vi "GET HARDWARE REFS CLUSTER.vi"(11 "HARDWARE cluster":T22 {"MOTORS"."Motor Controller" items=["SPARK", "Existing", "SD540", "TALON SRX", "VICTOR SP", "TALON SR", "JAGUAR", "VICTOR"]; "AIR"."PRESSURE"."warning HIGH" format="%.2f"; "AIR"."PRESSURE"."warning LOW" format="%.2f"; "AIR"."PRESSURE"."nominal value" format="%.2f"; "DRIVE MOTORS"."Motor Controller" items=["SPARK", "Existing", "SD540", "TALON SRX", "VICTOR SP", "TALON SR", "JAGUAR", "VICTOR"]}) -> (1 "REF OUTPUT":cluster{T12[], T16[], T17[]}, 2 "REF INPUT":cluster{T1[], T3[], T7[], T9[], T10[]}, 3 "REF DRIVE JOYSTICK":T21)   [LabVIEW 2017]
uses:
  Controls/def HARDWARE CTRL info.ctl
  Controls/def MOTOR info.ctl
  Controls/ctrl MOTOR CTRLR SELECT.ctl
  <vilib>/Rock Robotics/SystemInterfaces/DIO/FPGA_DIOPWMChannel.ctl
  Controls/def USER CONTROL info.ctl
  <vilib>/Rock Robotics/WPI/Joystick/WPI_JoystickDeviceEnum.ctl
  Controls/def ENCODER info.ctl
  <vilib>/Rock Robotics/SystemInterfaces/DIO/FPGA_DIOChannel.ctl
  <vilib>/Rock Robotics/WPI/Encoder/WPI_EncoderType.ctl
  Controls/def GYRO info.ctl
  <vilib>/Rock Robotics/SystemInterfaces/spilib/spi_bus.ctl
  Controls/ctrl ANALOG CHANNEL SELECT.ctl
  Controls/def AIR PRESSURE info.ctl
  <vilib>/Rock Robotics/SystemInterfaces/AI/FPGA_AIChannel.ctl
  Controls/def COMPRESSOR info.ctl
  Controls/def SOLENOID info.ctl
  <vilib>/Rock Robotics/WPI/Solenoid/WPI_SolenoidChannel.ctl
  <vilib>/Rock Robotics/WPI/Solenoid/WPI_SolenoidValue.ctl
  Controls/def SERVO info.ctl
  Controls/def SONAR info.ctl
  Controls/ctrl SONAR DEVICE SELECT.ctl
  <vilib>/Rock Robotics/WPI/Ultrasonic/WPI_UltrasonicRangeUnits.ctl
  Controls/def RELAY info.ctl
  <vilib>/Rock Robotics/SystemInterfaces/DIO/FPGA_DIORelayChannel.ctl
  <vilib>/Rock Robotics/WPI/Relay/WPI_RelayDirection.ctl
  <vilib>/Rock Robotics/WPI/Relay/WPI_RelayValue.ctl
  Controls/def LIMIT SWITCH info.ctl
  <vilib>/Rock Robotics/WPI/Joystick/WPI_JoystickDevRef.ctl
  <vilib>/Rock Robotics/WPI/RobotDrive/WPI_RobotDriveDevRef.ctl
  <vilib>/Rock Robotics/WPI/MotorControl/WPI_MotorControlDeviceRef.ctl
  <vilib>/Rock Robotics/WPI/MotorControl/WPI_MotorControlType.ctl
  <vilib>/Rock Robotics/WPI/PWM/WPI_PWMDeadband.ctl
  <vilib>/Rock Robotics/WPI/PWM/Servo/WPI_ServoDeviceRef.ctl
  <vilib>/Rock Robotics/WPI/Relay/WPI_RelayDevRef.ctl
  <vilib>/Rock Robotics/WPI/Encoder/WPI_EncoderDevRef.ctl
  <vilib>/Rock Robotics/SystemInterfaces/Encoder/FPGA_EncoderIdx.ctl
  <vilib>/Rock Robotics/SystemInterfaces/Counter/FPGA_CounterCtrSystemIndex.ctl
  <vilib>/Rock Robotics/WPI/Ultrasonic/WPI_UltrasonicDeviceRef.ctl
  <vilib>/Rock Robotics/WPI/Switch/WPI_SwitchDevRef.ctl
  <vilib>/Rock Robotics/WPI/AnalogChannel/WPI_AnalogChannelDevRef.ctl
  Controls/ctrl MOTOR SELECT.ctl
  Controls/ctrl SERVO SELECT.ctl
  Controls/ctrl AIRPRESS SELECT.ctl
  Controls/ctrl SONAR SELECT.ctl
  Controls/ctrl ENCODER SELECT.ctl
  <vilib>/Rock Robotics/WPI/Utilities/WPI_GetSetVariantRefNum.vi
  <vilib>/Rock Robotics/WPI/Ultrasonic/WPI_SonarSRF04DigitalRefNum Registry Get.vi
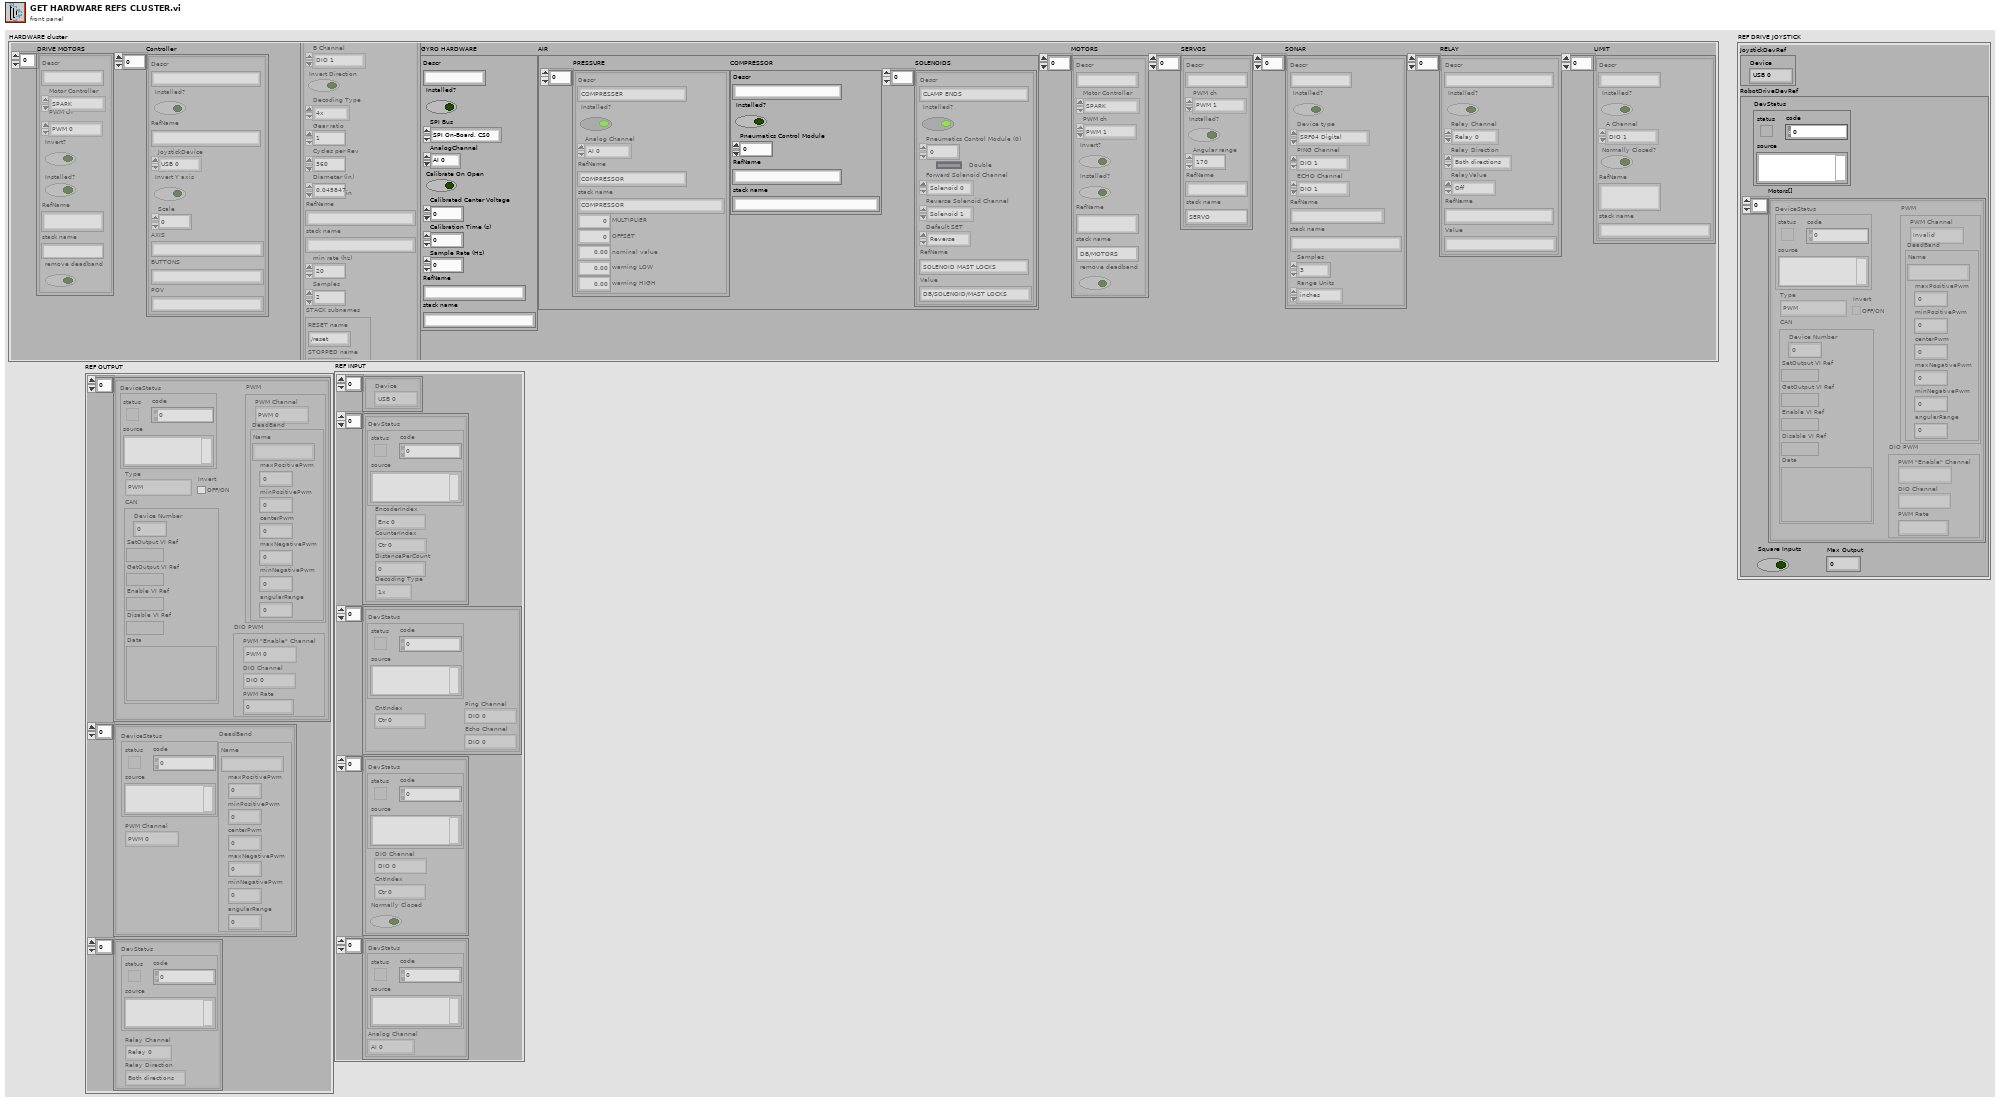
[diagram p1: front panel]
types:
  T1 = typedef "WPI_JoystickDevRef.ctl" = cluster{"Device":T2}
  T2 = typedef "WPI_JoystickDeviceEnum.ctl" = enum16{"USB 0", "USB 1", "USB 2", "USB 3", "USB 4", "USB 5"}
  T3 = typedef "WPI_EncoderDevRef.ctl" = cluster{"DevStatus":errorcluster, "EncoderIndex":T4, "CounterIndex":T5, "DistancePerCount":dbl, "Decoding Type":T6}
  T4 = typedef "FPGA_EncoderIdx.ctl" = enum8{"Enc 0", "Enc 1", "Enc 2", "Enc 3", "Enc 4", "Enc 5", "Enc 6", "Enc 7", "Invalid"}
  T5 = typedef "FPGA_CounterCtrSystemIndex.ctl" = enum8{"Ctr 0", "Ctr 1", "Ctr 2", "Ctr 3", "Ctr 4", "Ctr 5", "Ctr 6", "Ctr 7", "Invalid"}
  T6 = typedef "WPI_EncoderType.ctl" = enum16{"1x", "2x", "4x"}
  T7 = typedef "WPI_UltrasonicDeviceRef.ctl" = cluster{"DevStatus":errorcluster, "Ping Channel":T8, "Echo Channel":T8, "CntIndex":T5}
  T8 = typedef "FPGA_DIOChannel.ctl" = enum8{"DIO 0", "DIO 1", "DIO 2", "DIO 3", "DIO 4", "DIO 5", "DIO 6", "DIO 7", "DIO 8", "DIO 9", "DIO MXP 0", "DIO MXP 1", "DIO MXP 2", "DIO MXP 3", "DIO MXP 4", "DIO MXP 5", "DIO MXP 6", "DIO MXP 7", "DIO MXP 8", "DIO MXP 9", "DIO MXP 10", "DIO MXP 11", "DIO MXP 12", "DIO MXP 13", "DIO MXP 14", "DIO MXP 15", "SPI Port CS1", "SPI Port CS2", "SPI Port CS3", "SPI Port MISO", "SPI Port MOSI", "Invalid"}
  T9 = typedef "WPI_SwitchDevRef.ctl" = cluster{"DevStatus":errorcluster, "DIO Channel":T8, "CntIndex":T5, "Normally Closed":bool}
  T10 = typedef "WPI_AnalogChannelDevRef.ctl" = cluster{"DevStatus":errorcluster, "Analog Channel":T11}
  T11 = typedef "FPGA_AIChannel.ctl" = enum8{"AI 0", "AI 1", "AI 2", "AI 3", "AI MXP 0", "AI MXP 1", "AI MXP 2", "AI MXP 3", "Invalid"}
  T12 = typedef "WPI_MotorControlDeviceRef.ctl" = cluster{"DeviceStatus":errorcluster, "Type":T13, "PWM":cluster{"PWM Channel":T14, "DeadBand":T15}, "CAN":cluster{"Device Number":u8, "SetOutput VI Ref":variant, "GetOutput VI Ref":variant, "Enable VI Ref":variant, "Disable VI Ref":variant, "Data":variant}, "Invert":bool, "DIO PWM":cluster{"PWM \"Enable\" Channel":T14, "DIO Channel":T8, "PWM Rate":dbl}}
  T13 = typedef "WPI_MotorControlType.ctl" = enum16{"PWM", "CAN", "DIO PWM"}
  T14 = typedef "FPGA_DIOPWMChannel.ctl" = enum8{"PWM 0", "PWM 1", "PWM 2", "PWM 3", "PWM 4", "PWM 5", "PWM 6", "PWM 7", "PWM 8", "PWM 9", "PWM MXP 0", "PWM MXP 1", "PWM MXP 2", "PWM MXP 3", "PWM MXP 4", "PWM MXP 5", "PWM MXP 6", "PWM MXP 7", "PWM MXP 8", "PWM MXP 9", "Invalid"}
  T15 = typedef "WPI_PWMDeadband.ctl" = cluster{"Name":string, "maxPositivePwm":i32, "minPositivePwm":i32, "centerPwm":i32, "maxNegativePwm":i32, "minNegativePwm":i32, "angularRange":u16}
  T16 = typedef "WPI_ServoDeviceRef.ctl" = cluster{"DeviceStatus":errorcluster, "PWM Channel":T14, "DeadBand":T15}
  T17 = typedef "WPI_RelayDevRef.ctl" = cluster{"DevStatus":errorcluster, "Relay Channel":T18, "Relay Direction":T19}
  T18 = typedef "FPGA_DIORelayChannel.ctl" = enum8{"Relay 0", "Relay 1", "Relay 2", "Relay 3", "Invalid"}
  T19 = typedef "WPI_RelayDirection.ctl" = enum16{"Both directions", "Forward only", "Reverse only"}
  T20 = typedef "WPI_RobotDriveDevRef.ctl" = cluster{"DevStatus":errorcluster, "Motors[]":T12[], "Square Inputs":bool, "Max Output":dbl}
  T21 = cluster{"JoystickDevRef":T1, "RobotDriveDevRef":T20}
  T22 = typedef "def HARDWARE CTRL info.ctl" = cluster{"DRIVE MOTORS":T23[], "Controller":T25[], "ENCODERS":T26[], "GYRO HARDWARE":T27, "AIR":cluster{"PRESSURE":T30[], "COMPRESSOR":T31, "SOLENOIDS":T32[]}, "MOTORS":T23[], "SERVOS":T35[], "SONAR":T36[], "RELAY":T39[], "LIMIT":T41[]}
  T23 = typedef "def MOTOR info.ctl" = cluster{"Descr":string, "Motor Controller":T24, "PWM ch":T14, "Invert?":bool, "Installed?":bool, "RefName":string, "stack name":string, "remove deadband":bool}
  T24 = typedef "ctrl MOTOR CTRLR SELECT.ctl" = u16
  T25 = typedef "def USER CONTROL info.ctl" = cluster{"Descr":string, "Installed?":bool, "RefName":string, "JoystickDevice":T2, "Invert Y axis":bool, "Scale":dbl, "AXIS":string, "BUTTONS":string, "POV":string}
  T26 = typedef "def ENCODER info.ctl" = cluster{"Descr":string, "Installed?":bool, "A Channel":T8, "B Channel":T8, "Invert Direction":bool, "Enum":T6, "Gear ratio":dbl, "Cycles per Rev":dbl, "Diameter (in)":dbl[unit], "RefName":string, "stack name":string, "min rate (hz)":dbl, "Samples":u8, "STACK subnames":cluster{"RESET name":string, "STOPPED name":string, "DIRECTION name":string, "RATE name":string, "INSTALLED name":string}}
  T27 = typedef "def GYRO info.ctl" = cluster{"Descr":string, "Installed?":bool, "SPI Bus":T28, "AnalogChannel":T29, "Calibrate On Open":bool, "Calibrated Center Voltage":dbl, "Calibration Time (s)":dbl, "Sample Rate (Hz)":dbl, "RefName":string, "stack name":string}
  T28 = typedef "spi_bus.ctl" = enum16{"SPI On-Board, CS0", "SPI On-Board, CS1", "SPI On-Board, CS2", "SPI On-Board, CS3", "SPI MXP", "Invalid"}
  T29 = typedef "ctrl ANALOG CHANNEL SELECT.ctl" = enum8{"AI 0", "AI 1", "Invalid"}
  T30 = typedef "def AIR PRESSURE info.ctl" = cluster{"Descr":string, "Installed?":bool, "Channel":T11, "RefName":string, "stack name":string, "MULTIPLIER":dbl, "OFFSET":dbl, "nominal value":dbl, "warning LOW":dbl, "warning HIGH":dbl}
  T31 = typedef "def COMPRESSOR info.ctl" = cluster{"Descr":string, "Installed?":bool, "Pneumatics Control Module":u8, "RefName":string, "stack name":string}
  T32 = typedef "def SOLENOID info.ctl" = cluster{"Descr":string, "Installed?":bool, "Pneumatics Control Module (0)":u8, "DBL":bool, "SolenoidChannel":T33, "SolenoidChannel":T33, "Default SET":T34, "RefName":string, "Value":string}
  T33 = typedef "WPI_SolenoidChannel.ctl" = enum8{"Solenoid 0", "Solenoid 1", "Solenoid 2", "Solenoid 3", "Solenoid 4", "Solenoid 5", "Solenoid 6", "Solenoid 7", "Invalid"}
  T34 = typedef "WPI_SolenoidValue.ctl" = enum16{"Off", "On", "Forward", "Reverse"}
  T35 = typedef "def SERVO info.ctl" = cluster{"Descr":string, "PWM ch":T14, "Installed?":bool, "Angular range":dbl, "RefName":string, "stack name":string}
  T36 = typedef "def SONAR info.ctl" = cluster{"Descr":string, "Installed?":bool, "Device type":T37, "PING Channel":T8, "ECHO Channel":T8, "RefName":string, "stack name":string, "Samples":i32, "Range Units":T38}
  T37 = typedef "ctrl SONAR DEVICE SELECT.ctl" = enum16{"SRF04 Digital", "MB1010 Digital", "MB1010 Analog", "SRF08 Digital"}
  T38 = typedef "WPI_UltrasonicRangeUnits.ctl" = enum16{"inches", "mm"}
  T39 = typedef "def RELAY info.ctl" = cluster{"Descr":string, "Installed?":bool, "RelayChannel":T18, "Relay Direction":T19, "Relay Value":T40, "RefName":string, "Value":string}
  T40 = typedef "WPI_RelayValue.ctl" = enum16{"Off", "On", "Forward", "Reverse"}
  T41 = typedef "def LIMIT SWITCH info.ctl" = cluster{"Descr":string, "Installed?":bool, "A Channel":T8, "Normally Closed?":bool, "RefName":string, "stack name":string}
  T42 = typedef "ctrl ENCODER SELECT.ctl" = u16
  T43 = typedef "ctrl SONAR SELECT.ctl" = u16
  T44 = typedef "ctrl AIRPRESS SELECT.ctl" = u16
  T45 = typedef "ctrl MOTOR SELECT.ctl" = u16
  T46 = typedef "ctrl SERVO SELECT.ctl" = u16
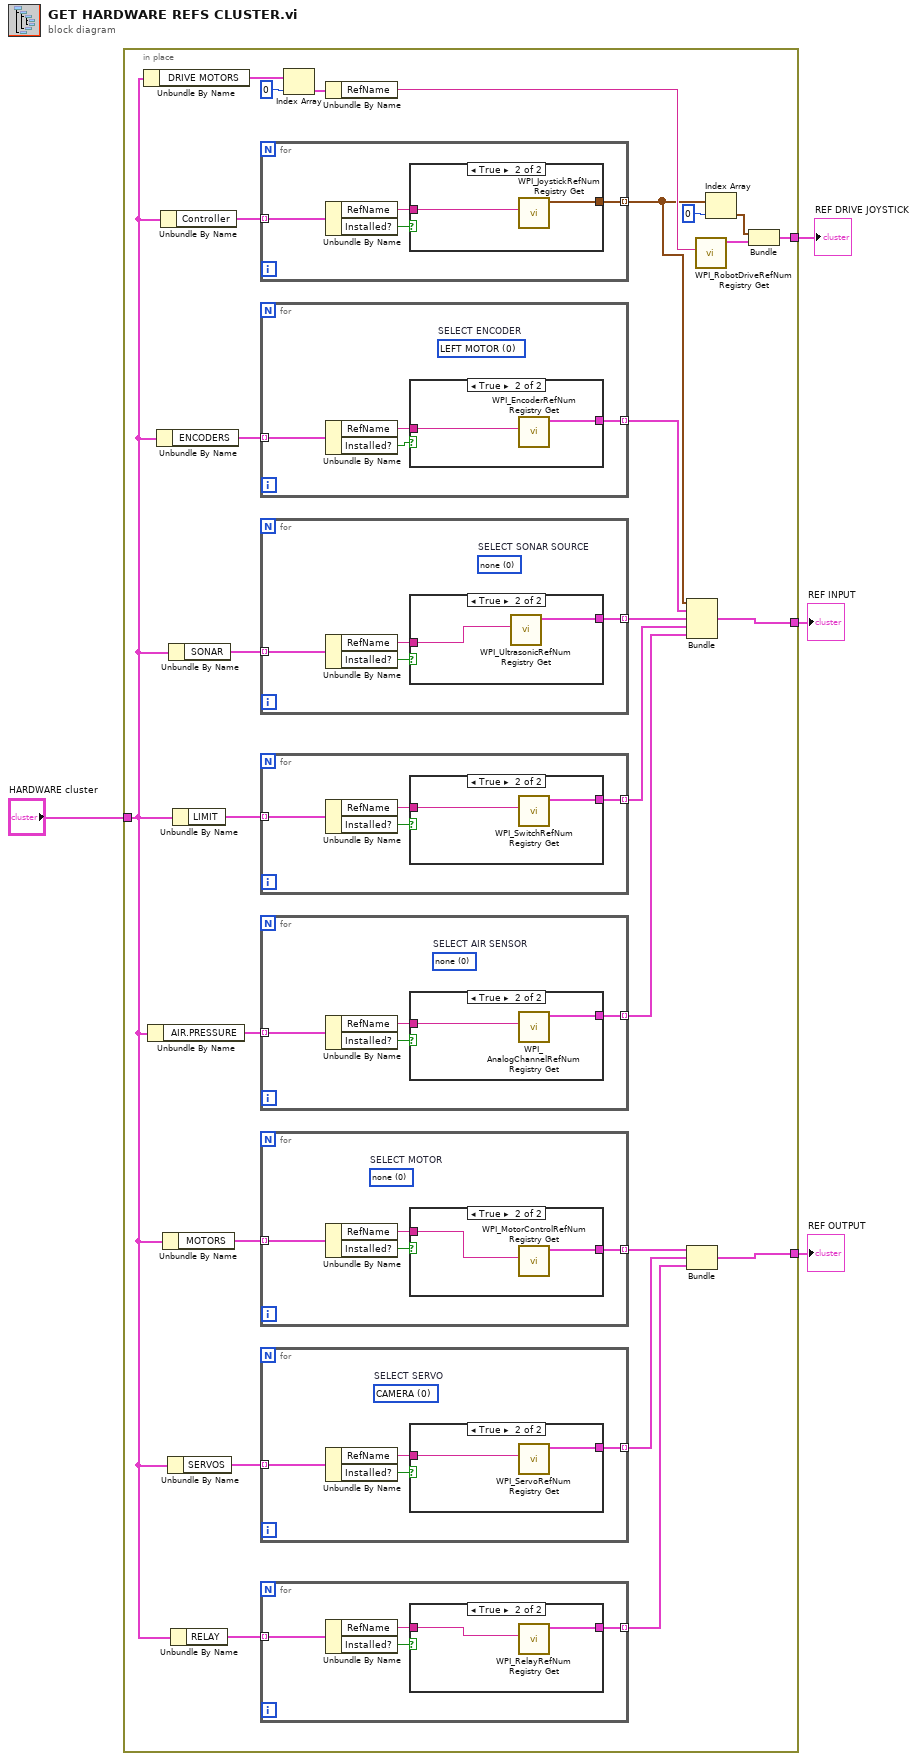
[diagram p0: block diagram]
diagram:
  n1 = in-place {
    in-place-border: [w26] -> w3
    in-place-border: "HARDWARE cluster" -> [w8]
    in-place-border: [w17] -> w1
    in-place-border: [w10] -> w2
    n2 = Unbundle By Name(w8) -> ("DRIVE MOTORS"=w30:T23[])
    n3 = Unbundle By Name(w8) -> ("AIR.PRESSURE"=w22:T30[])
    n4 = Unbundle By Name(w8) -> ("ENCODERS"=w25:T26[])
    n5 = Unbundle By Name(w8) -> ("Controller"=w9:T25[])
    n6 = Unbundle By Name(w8) -> ("MOTORS"=w20:T23[])
    n7 = Unbundle By Name(w8) -> ("SERVOS"=w21:T35[])
    n8 = Unbundle By Name(w8) -> ("SONAR"=w24:T36[])
    n9 = Unbundle By Name(w8) -> ("RELAY"=w19:T39[])
    n10 = Unbundle By Name(w8) -> ("LIMIT"=w23:T41[])
    n11 = for {
      tunnel: w9 -> [w35] mode=indexing
      tunnel: [w33] -> w5 mode=indexing
      n12 = Unbundle By Name(w35) -> ("RefName"=w34:string, "Installed?"=w32:bool)
      n13 = case shown="True" w32 {
        tunnel: w34 -> [_ w37]
        tunnel: [_ w36] -> w33
        frame False {
        }
        frame True {
          n14 = call <vilib>:"WPI_JoystickRefNum Registry Get.vi"("refnum name"=w37) -> ("JoystickDevRef"=w36:T1)  [unwired: 9 in, 1 out]
        }
      }
    }
    n15 = for {
      tunnel: w25 -> [w77] mode=indexing
      tunnel: [w75] -> w18 mode=indexing
      (unwired) T42 0 items=["LEFT MOTOR", "RIGHT MOTOR"]  # SELECT ENCODER
      n16 = Unbundle By Name(w77) -> ("RefName"=w76:string, "Installed?"=w74:bool)
      n17 = case shown="True" w74 {
        tunnel: w76 -> [_ w79]
        tunnel: [_ w78] -> w75
        frame False {
        }
        frame True {
          n18 = call <vilib>:"WPI_EncoderRefNum Registry Get.vi"("refnum name"=w79) -> ("EncoderDevRef"=w78:T3)  [unwired: 9 in, 1 out]
        }
      }
    }
    n19 = for {
      tunnel: w24 -> [w71] mode=indexing
      tunnel: [w69] -> w16 mode=indexing
      (unwired) T43 0 items=["none"]  # SELECT SONAR SOURCE
      n20 = Unbundle By Name(w71) -> ("RefName"=w70:string, "Installed?"=w68:bool)
      n21 = case shown="True" w68 {
        tunnel: w70 -> [_ w73]
        tunnel: [_ w72] -> w69
        frame False {
        }
        frame True {
          n22 = call-poly <vilib>:"WPI_UltrasonicRefNum Registry Get.vi"("refnum name"=w73) -> ("SonarSRF04DevRef"=w72:T7)  [unwired: 9 in, 1 out]
        }
      }
    }
    n23 = for {
      tunnel: w23 -> [w65] mode=indexing
      tunnel: [w63] -> w15 mode=indexing
      n24 = Unbundle By Name(w65) -> ("RefName"=w64:string, "Installed?"=w62:bool)
      n25 = case shown="True" w62 {
        tunnel: w64 -> [_ w67]
        tunnel: [_ w66] -> w63
        frame False {
        }
        frame True {
          n26 = call <vilib>:"WPI_SwitchRefNum Registry Get.vi"("refnum name"=w67) -> ("SwitchDevRef"=w66:T9)  [unwired: 9 in, 1 out]
        }
      }
    }
    n27 = for {
      tunnel: w22 -> [w59] mode=indexing
      tunnel: [w57] -> w14 mode=indexing
      (unwired) T44 0 items=["none"]  # SELECT AIR SENSOR
      n28 = Unbundle By Name(w59) -> ("RefName"=w58:string, "Installed?"=w56:bool)
      n29 = case shown="True" w56 {
        tunnel: w58 -> [_ w61]
        tunnel: [_ w60] -> w57
        frame False {
        }
        frame True {
          n30 = call <vilib>:"WPI_AnalogChannelRefNum Registry Get.vi"("refnum name"=w61) -> ("AIDeviceRef"=w60:T10)  [unwired: 9 in, 1 out]
        }
      }
    }
    n31 = for {
      tunnel: w20 -> [w47] mode=indexing
      tunnel: [w45] -> w13 mode=indexing
      (unwired) T45 0 items=["none"]  # SELECT MOTOR
      n32 = Unbundle By Name(w47) -> ("RefName"=w46:string, "Installed?"=w44:bool)
      n33 = case shown="True" w44 {
        tunnel: w46 -> [_ w49]
        tunnel: [_ w48] -> w45
        frame False {
        }
        frame True {
          n34 = call <vilib>:"WPI_MotorControlRefNum Registry Get.vi"("refnum name"=w49) -> ("MotorControlDevRef"=w48:T12)  [unwired: 9 in, 1 out]
        }
      }
    }
    n35 = for {
      tunnel: w21 -> [w53] mode=indexing
      tunnel: [w51] -> w12 mode=indexing
      (unwired) T46 0 items=["CAMERA", "SHOOTER", "BALL AGITATOR"]  # SELECT SERVO
      n36 = Unbundle By Name(w53) -> ("RefName"=w52:string, "Installed?"=w50:bool)
      n37 = case shown="True" w50 {
        tunnel: w52 -> [_ w55]
        tunnel: [_ w54] -> w51
        frame False {
        }
        frame True {
          n38 = call <vilib>:"WPI_ServoRefNum Registry Get.vi"("refnum name"=w55) -> ("ServoDeviceRef"=w54:T16)  [unwired: 9 in, 1 out]
        }
      }
    }
    n39 = for {
      tunnel: w19 -> [w41] mode=indexing
      tunnel: [w39] -> w11 mode=indexing
      n40 = Unbundle By Name(w41) -> ("RefName"=w40:string, "Installed?"=w38:bool)
      n41 = case shown="True" w38 {
        tunnel: w40 -> [_ w43]
        tunnel: [_ w42] -> w39
        frame False {
        }
        frame True {
          n42 = call <vilib>:"WPI_RelayRefNum Registry Get.vi"("refnum name"=w43) -> ("RelayDevRef"=w42:T17)  [unwired: 9 in, 1 out]
        }
      }
    }
    n43 = Index Array(array=w30, index=0) -> (element=w28:T23)
    n44 = Unbundle By Name(w28) -> ("RefName"=w27:string)
    n45 = Bundle(w5, w18, w16, w15, w14) -> (w17:cluster{T1[], T3[], T7[], T9[], T10[]})  [unwired: 1 in]
    n46 = Bundle(w13, w12, w11) -> (w10:cluster{T12[], T16[], T17[]})  [unwired: 1 in]
    n47 = call <vilib>:"WPI_RobotDriveRefNum Registry Get.vi"("refnum name"=w27) -> ("RobotDriveDevRef"=w31:T20)  [unwired: 1 in, 9 out]
    n48 = Index Array(array=w5, index=0) -> (element=w6:T1)
    n49 = Bundle("JoystickDevRef"=w6, "RobotDriveDevRef"=w31) -> (w26:T21)  [unwired: 1 out]
  }
  "REF DRIVE JOYSTICK" <- w3
  "REF OUTPUT" <- w2
  "REF INPUT" <- w1
